vi "sum of 2 Gaussians with offset.vi"(3 "output control":T1, 4 "data":variant, 5 "X":dbl[](array[numeric]), 6 "a":dbl[](array[numeric])) -> (0 "error out":errorcluster, 1 "f'(X,a)":dbl[][](array[numeric]), 2 "f(X,a)":dbl[](array[numeric]))   [LabVIEW 2015]
doc: "Sum of three Gaussians, plus DC offset."
uses:
  <vilib>/gmath/NumericalOptimization/LM_output select.ctl
  <vilib>/gmath/NI_Gmath.lvlib
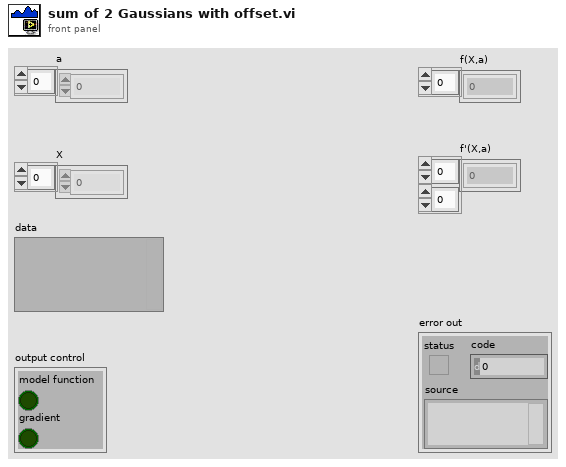
[diagram p1: front panel]
types:
  T1 = typedef "NI_Gmath.lvlib/LM_output select.ctl" = cluster{"model function":bool, "gradient":bool}
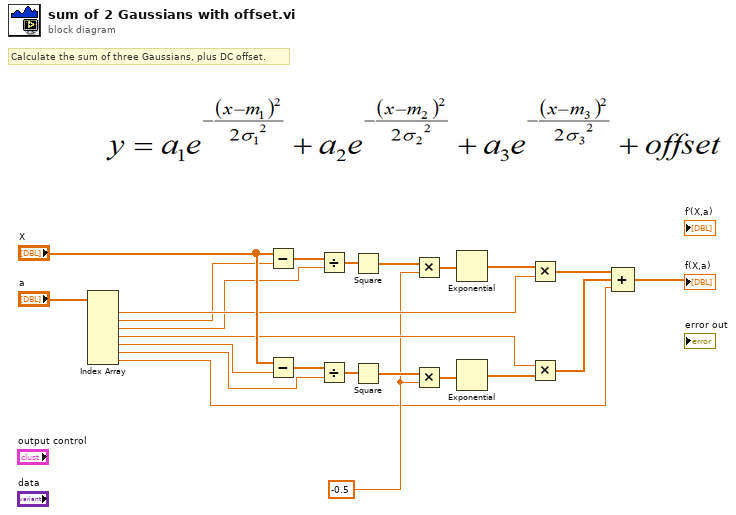
[diagram p0: block diagram]
diagram:
  w2 = -0.5
  # "Calculate the sum of three Gaussians, plus DC offset."
  n1 = Index Array(array="a") -> (element #1=w22:dbl, element #2=w21:dbl, element #3=w20:dbl, element #4=w19:dbl, element #5=w18:dbl, element #6=w17:dbl, element #7=w1:dbl)  [unwired: 7 in]
  n2 = Subtract(x="X", y=w21) -> (x-y=w6:dbl[])
  n3 = Subtract(x="X", y=w18) -> (x-y=w5:dbl[])
  n4 = Divide(x=w6, y=w20) -> (x/y=w14:dbl[])
  n5 = Divide(x=w5, y=w17) -> (x/y=w11:dbl[])
  n6 = Square(x=w14) -> (x^2=w4:dbl[])
  n7 = Square(x=w11) -> (x^2=w3:dbl[])
  n8 = Multiply(x=w4, y=w2) -> (x*y=w8:dbl[])
  n9 = Multiply(x=w3, y=w2) -> (x*y=w7:dbl[])
  n10 = Exponential(1:w8) -> (0:w13:dbl[])
  n11 = Exponential(1:w7) -> (0:w12:dbl[])
  n12 = Multiply(x=w13, y=w22) -> (x*y=w10:dbl[])
  n13 = Multiply(x=w19, y=w12) -> (x*y=w9:dbl[])
  n14 = Compound Arithmetic op=ADD(w10, w9, w1) -> (→"f(X,a)":dbl[])
